vi "7_nov.vi"() -> ()   [LabVIEW 2020]
uses:
  <instrlib>/Agilent B2900 Series/Public/Configure/Measurement/Configure Measurement (Resistance).vi
  <instrlib>/Agilent B2900 Series/Public/Data/Read Measurement Result (Single Point).vi
  <instrlib>/Agilent B2900 Series/Agilent B2900 Series.lvlib
panel:
  out "VISA resource name out":refnum<visa-resource-name>
  out "error out":errorcluster
  out "Measurement Result":dbl
  in  "Measurement Mode (0:Voltage)":enum16{"Voltage", "Current", "Resistance"}(ring)
  in  "Resistance Measurement Mode":i32(ring)=1 items=["Manual", "Auto"]
  in  "VISA resource name":refnum<visa-resource-name>="COM1"
  out "Measurement Result(ohms)":dbl
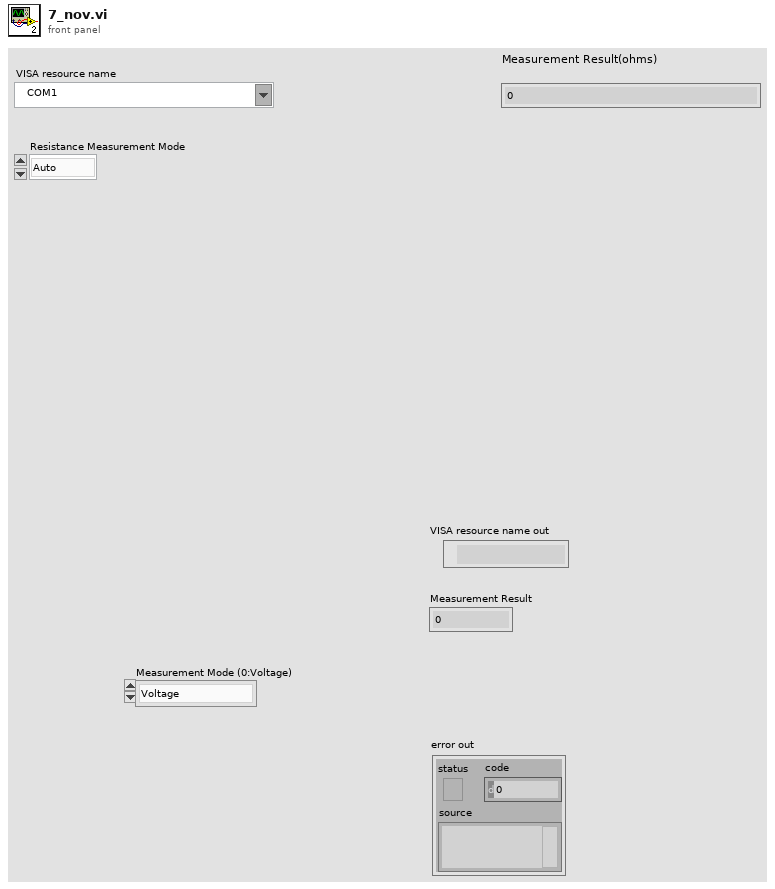
[diagram p1: front panel]
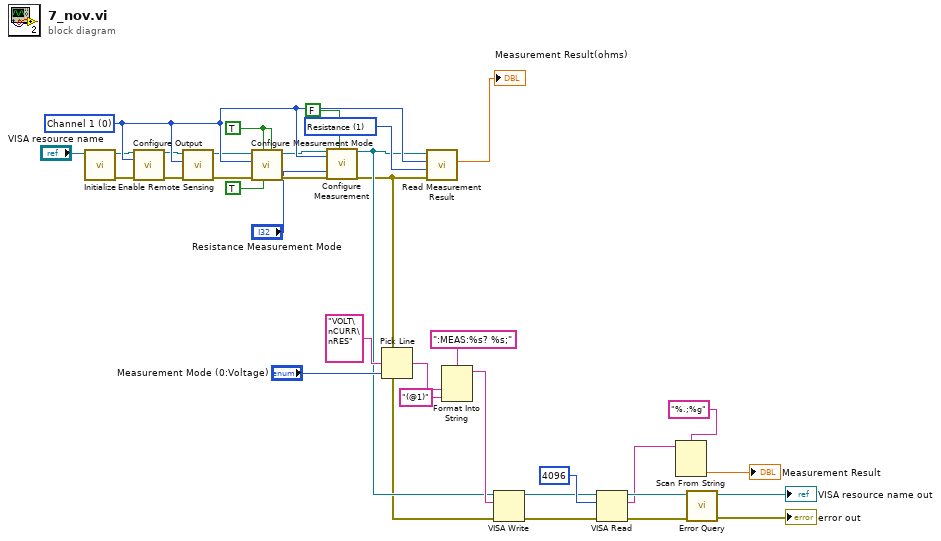
[diagram p0: block diagram]
diagram:
  w34 = 0 items=["Channel 1", "Channel 2"] ("Channel (0: Channel 1)")
  w32 = 1 items=["Current", "Resistance", "Source Output Setting", "Status", "Time", "Voltage"] ("Data Mode (5: Voltage)")
  w31 = TRUE ("Enable Voltage Measurement (T: Enable)")
  n1 = call <instrlib>:"Initialize.vi"("VISA resource name"="VISA resource name") -> ("error out"=w22:errorcluster, "VISA resource name out"=w23:refnum<visa-resource-name>)  [unwired: 9 in]
  n2 = call <instrlib>:"Configure Output.vi"("VISA resource name"=w23, "Channel (0: Channel 1)"=w34, "error in (no error)"=w22) -> ("VISA resource name out"=w27:refnum<visa-resource-name>, "error out"=w24:errorcluster)  [unwired: 11 in]
  n3 = call <instrlib>:"Enable Remote Sensing.vi"("error in (no error)"=w24, "Channel (0: Channel 1)"=w34, "VISA resource name"=w27) -> ("error out"=w25:errorcluster, "VISA resource name out"=w28:refnum<visa-resource-name>)  [unwired: 7 in]
  n4 = call <instrlib>:"Configure Measurement Mode.vi"("Enable Current Measurement (T: Enable)"=w31, "Enable Resistance Measurement (F: Disable)"=TRUE, "Enable Voltage Measurement (T: Enable)"=w31, "error in (no error)"=w25, "Channel (0: Channel 1)"=w34, "VISA resource name"=w28) -> ("error out"=w26:errorcluster, "VISA resource name out"=w29:refnum<visa-resource-name>)  [unwired: 4 in]
  n5 = call-poly <instrlib>:"Configure Measurement.vi"("VISA resource name"=w29, "Channel (0: Channel 1)"=w34, "Resistance Measurement Mode (1: Auto)"="Resistance Measurement Mode", "error in (no error)"=w26, "Enable Resistance Compensation (F: Disable)"=FALSE) -> ("VISA resource name out"=w2:refnum<visa-resource-name>, "error out"=w1:errorcluster)  [unwired: 13 in]
  n6 = Pick Line(multi-line string="VOLT\nCURR\nRES", line index="Measurement Mode (0:Voltage)") -> (output string=w6:string)  [unwired: 1 in]
  n7 = call-poly <instrlib>:"Read Measurement Result.vi"("error in (no error)"=w1, "Data Mode (5: Voltage)"=w32, "Channel (0: Channel 1)"=w34, "VISA resource name"=w2) -> ("Measurement Result"=→"Measurement Result(ohms)":dbl)  [unwired: 5 in, 2 out]
  n8 = Format Into String(format string=":MEAS:%s? %s;", w6, "(@1)" ("input 2")) -> (resulting string=w9:string)  [unwired: 2 in, 1 out]
  n9 = VISA Write(VISA resource name=w2, write buffer=w9, error in (no error)=w1) -> (VISA resource name out=w16:refnum<visa-resource-name>, error out=w15:errorcluster)  [unwired: 1 out]
  n10 = VISA Read(VISA resource name=w16, byte count=u32 4096, error in (no error)=w15) -> (VISA resource name out=w14:refnum<visa-resource-name>, read buffer=w3:string, error out=w13:errorcluster)  [unwired: 1 out]
  n11 = Scan From String(format string="%.;%g", input string=w3) -> (output 1=→"Measurement Result":dbl)  [unwired: 3 in, 3 out]
  n12 = call <instrlib>:"Error Query.vi"("error in (no error)"=w13, "VISA resource name"=w14) -> ("error out"=→"error out":errorcluster, "VISA resource name out"=→"VISA resource name out":refnum<visa-resource-name>)  [unwired: 6 in, 2 out]
